vi "全局 反控命令枚举.vi"() -> ()   [LabVIEW 2016, in "数据传输系统.lvlib"]
panel:
  out "是否判断反馈？":bool
  out "执行结果":u16
  out "执行反馈":bool
  in  "执行结果定义":u16(ring) items=["执行成功"=1, "执行失败，但不知道原因"=2, "命令请求条件错误"=3, "通讯超时"=4, "系统繁忙不能执行"=5, "系统故障"=6, "没有数据"=100]
  in  "反控命令枚举":enum16{"返回请求应答", "返回执行结果"}(ring)
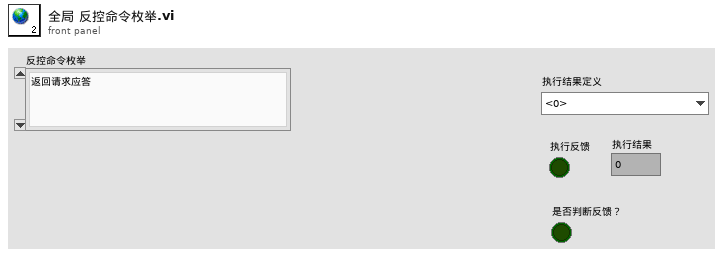
[diagram p1: front panel]
diagram:
